vi "Begin.vi"(8 "error in":errorcluster) -> (0 "error out":errorcluster)   [LabVIEW 2018]
doc: "Called before other user functions, this VI is expected to open initial I/O refnums, load in file data, and do all program initialization. Notice that the <B>error out</B> terminal is simply used for data flow. Wiring it to other structures or subVIs ensures that this VI runs first."
uses:
  <vilib>/Rock Robotics/WPI/DriverStation/WPI_DriverStationRobotMode2.ctl
  <vilib>/Rock Robotics/WPI/Joystick/WPI_JoystickDeviceEnum.ctl
  <vilib>/Rock Robotics/WPI/Solenoid/WPI_SolenoidChannel.ctl
  <vilib>/Rock Robotics/WPI/ThirdParty/Phoenix-LabVIEW/Motor Controller/Controls/CTRE_Phoenix_MotorControl_NeutralMode.ctl
  <vilib>/Rock Robotics/WPI/ThirdParty/REV Robotics/SPARK MAX/Typedef/Spark MAX Idle Mode.ctl
  2019 Deep Space Beta/Robot Global Data.vi
  <vilib>/Rock Robotics/Network Tables/NT Write String Array.vi
  <vilib>/Rock Robotics/WPI/Solenoid/WPI_SolenoidOpenDouble.vi
  <vilib>/Rock Robotics/WPI/Solenoid/WPI_SolenoidOpenSingle.vi
  <vilib>/Rock Robotics/WPI/Utilities/WPI_GetSetVariantRefNum.vi
  <vilib>/Rock Robotics/WPI/SerialPort/WPI_SerialPort.ctl
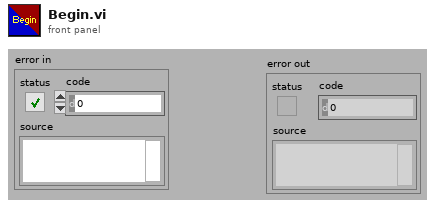
[diagram p1: front panel]
types:
  T1 = typedef "Spark MAX Idle Mode.ctl" = enum16{"Coast", "Brake"}
  T2 = typedef "CTRE_Phoenix_MotorControl_NeutralMode.ctl" = enum8{"EEPROMSetting", "Override to Coast", "Override to Brake"}
  T3 = typedef "WPI_SolenoidChannel.ctl" = enum8{"Solenoid 0", "Solenoid 1", "Solenoid 2", "Solenoid 3", "Solenoid 4", "Solenoid 5", "Solenoid 6", "Solenoid 7", "Invalid"}
  T4 = typedef "WPI_JoystickDeviceEnum.ctl" = enum16{"USB 0", "USB 1", "USB 2", "USB 3", "USB 4", "USB 5"}
  T5 = typedef "WPI_DriverStationRobotMode2.ctl" = enum16{"Autonomous Disabled", "Autonomous Enabled", "Teleop Disabled", "Teleop Enabled", "Disconnected", "Finish", "Test Disabled", "Test Enabled", "Emergency Stopped"}
  T6 = typedef "WPI_JoystickDevRef.ctl" = cluster{"Device":T4}
  T7 = typedef "WPI_MotorControlDeviceRef.ctl" = cluster{"DeviceStatus":errorcluster, "Type":T8, "PWM":cluster{"PWM Channel":T9, "DeadBand":T10}, "CAN":cluster{"Device Number":u8, "SetOutput VI Ref":variant, "GetOutput VI Ref":variant, "Enable VI Ref":variant, "Disable VI Ref":variant, "Data":variant}, "Invert":bool, "DIO PWM":cluster{"PWM \"Enable\" Channel":T9, "DIOChannel":T11, "PWM Rate":dbl}}
  T8 = typedef "WPI_MotorControlType.ctl" = enum16{"PWM", "CAN", "DIO PWM"}
  T9 = typedef "FPGA_DIOPWMChannel.ctl" = enum8{"PWM 0", "PWM 1", "PWM 2", "PWM 3", "PWM 4", "PWM 5", "PWM 6", "PWM 7", "PWM 8", "PWM 9", "PWM MXP 0", "PWM MXP 1", "PWM MXP 2", "PWM MXP 3", "PWM MXP 4", "PWM MXP 5", "PWM MXP 6", "PWM MXP 7", "PWM MXP 8", "PWM MXP 9", "Invalid"}
  T10 = typedef "WPI_PWMDeadband.ctl" = cluster{"Name":string, "maxPositivePwm":i32, "minPositivePwm":i32, "centerPwm":i32, "maxNegativePwm":i32, "minNegativePwm":i32, "angularRange":u16}
  T11 = typedef "FPGA_DIOChannel.ctl" = enum8{"DIO 0", "DIO 1", "DIO 2", "DIO 3", "DIO 4", "DIO 5", "DIO 6", "DIO 7", "DIO 8", "DIO 9", "DIO MXP 0", "DIO MXP 1", "DIO MXP 2", "DIO MXP 3", "DIO MXP 4", "DIO MXP 5", "DIO MXP 6", "DIO MXP 7", "DIO MXP 8", "DIO MXP 9", "DIO MXP 10", "DIO MXP 11", "DIO MXP 12", "DIO MXP 13", "DIO MXP 14", "DIO MXP 15", "SPI Port CS1", "SPI Port CS2", "SPI Port CS3", "SPI Port MISO", "SPI Port MOSI", "Invalid"}
  T12 = typedef "WPI_SerialPort.ctl" = enum16{"Onboard RS-232", "MXP TTL", "USB 1", "USB 2"}
  T13 = typedef "WPI_SerialPortRef.ctl" = cluster{"DevStatus":errorcluster, "Serial Port Name":refnum<visa-resource-name>}
  T14 = typedef "WPI_CompressorDevRef.ctl" = cluster{"DevStatus":errorcluster, "Pneumatics Control Module":u8}
  T15 = typedef "WPI_SolenoidDevRef.ctl" = cluster{"DevStatus":errorcluster, "Pneumatics Control Module":u8, "Forward Solenoid Channel":T3, "Reverse Solenoid Channel":T3}
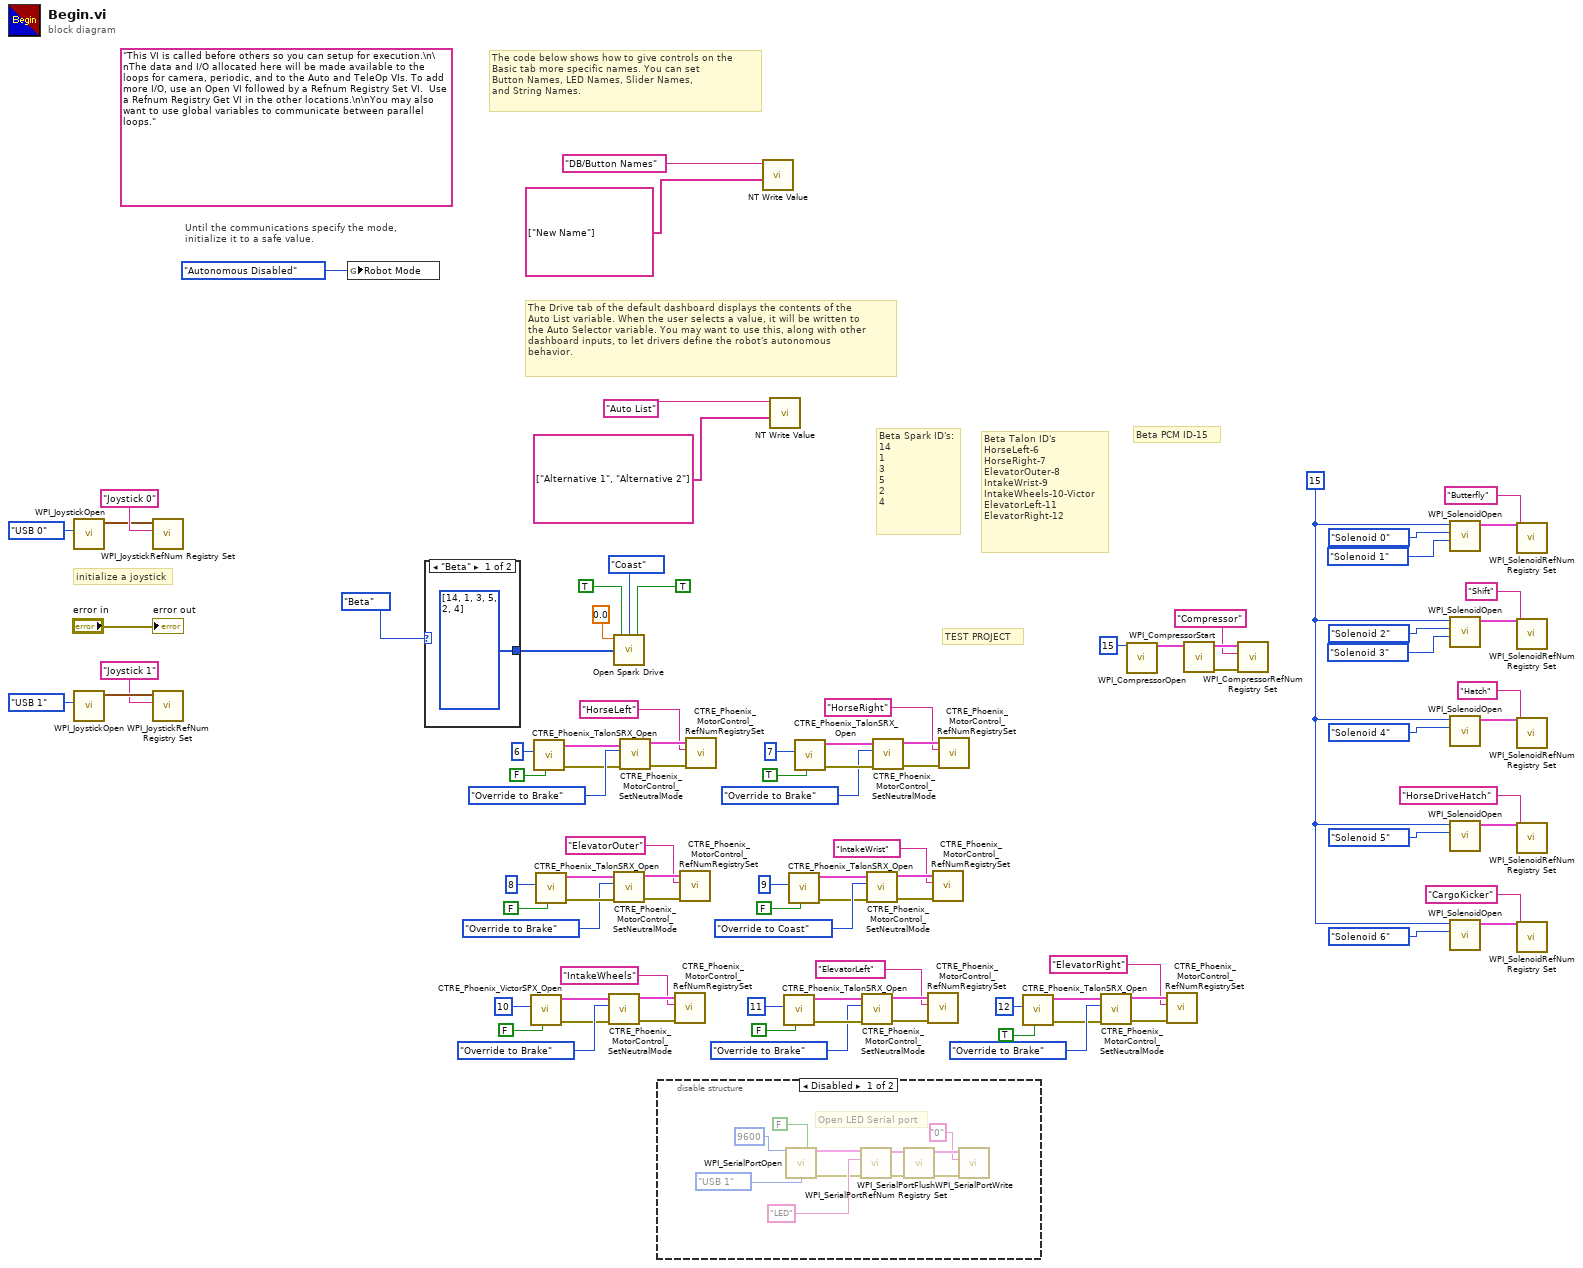
[diagram p0: block diagram]
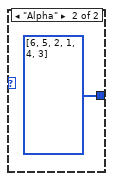
[diagram p2: hidden frame]
diagram:
  w69 = u8 15 ("Pneumatics Control Module (0)")
  (unwired) "This VI is called before others so you can setup for execution.\n\nThe data and I/O allocated here will be made available to the loops for camera, periodic, and to the Auto and TeleOp VIs. To add more I/O, use an Open VI followed by a Refnum Registry Set VI.  Use a Refnum Registry Get VI in the other locations.\n\nYou may also want to use global variables to communicate between parallel loops."
  # "Beta PCM ID-15"
  # "Beta Talon ID's\nHorseLeft-6\nHorseRight-7\nElevatorOuter-8\nIntakeWrist-9\nIntakeWheels-10-Victor\nElevatorLeft-11\nElevatorRight-12"
  # "Beta Spark ID's:\n14\n1\n3\n5\n2\n4"
  # "TEST PROJECT"
  # "The Drive tab of the default dashboard displays the contents of the\nAuto List variable. When the user selects a value, it will be written to\nthe Auto Selector variable. You may want to use this, along with other\ndashboard inputs, to let drivers define the robot's autonomous\nbehavior."
  # "The code below shows how to give controls on the\nBasic tab more specific names. You can set\nButton Names, LED Names, Slider Names,\nand String Names."
  # "initialize a joystick"
  # "Until the communications specify the mode,\ninitialize it to a safe value."
  n1 = call <vilib>:"WPI_JoystickOpen.vi"("JoystickDevice"=WPI_JoystickDeviceEnum."USB 0") -> ("JoystickDevRef"=w95:T6)  [unwired: 10 in]
  n2 = call <vilib>:"WPI_JoystickOpen.vi"("JoystickDevice"=WPI_JoystickDeviceEnum."USB 1") -> ("JoystickDevRef"=w87:T6)  [unwired: 10 in]
  n3 = call <vilib>:"WPI_JoystickRefNum Registry Set.vi"("refnum name"="Joystick 0", "JoystickDevRef"=w95) -> ()  [unwired: 8 in, 2 out]
  n4 = call <vilib>:"WPI_JoystickRefNum Registry Set.vi"("refnum name"="Joystick 1", "JoystickDevRef"=w87) -> ()  [unwired: 8 in, 2 out]
  n5 = global write "Robot Global Data.vi" "Robot Mode"(WPI_DriverStationRobotMode2."Autonomous Disabled" ("Robot Mode")) -> ()
  n6 = case shown="\"Beta\"" enum16{"Alpha", "Beta"}."Beta" {
    tunnel: [u8[] [14, 1, 3, 5, 2, 4] ("CAN IDs") u8[] [6, 5, 2, 1, 4, 3] ("CAN IDs")] -> w1
    frame "Beta" {
    }
    frame "Alpha" {
    }
  }
  n7 = call <vilib>:"CTRE_Phoenix_VictorSPX_Open.vi"("Invert"=FALSE, "Device Number"=u8 10) -> ("error out"=w50:errorcluster, "CAN Talon SRX Ref"=w51:T7)  [unwired: 8 in]
  n8 = call <vilib>:"CTRE_Phoenix_TalonSRX_Open.vi"("Invert"=FALSE, "Device Number"=u8 6) -> ("error out"=w16:errorcluster, "CAN Talon SRX Ref"=w17:T7)  [unwired: 8 in]
  n9 = call <vilib>:"CTRE_Phoenix_TalonSRX_Open.vi"("Invert"=FALSE, "Device Number"=u8 8) -> ("error out"=w55:errorcluster, "CAN Talon SRX Ref"=w54:T7)  [unwired: 8 in]
  n10 = call <vilib>:"CTRE_Phoenix_MotorControl_SetNeutralMode.vi"("error in (no error)"=w50, "Motor Control Neutral Mode"=CTRE_Phoenix_MotorControl_NeutralMode."Override to Brake", "PhoenixMotorControlDevRef"=w51) -> ("error out"=w48:errorcluster, "PhoenixMotorControlDevRef"=w49:T7)  [unwired: 7 in]
  n11 = call "Open Spark Drive.vi"("Set Master/Slave?"=TRUE, "Set Ramp Rate?"=TRUE, "CAN IDs"=w1, "Idle Mode"=Spark_MAX_Idle_Mode."Coast", "Full Acceleration Time"=sgl 0.0 ("Seconds from neutral to full (0)")) -> ()  [unwired: 7 in]
  n12 = call <vilib>:"CTRE_Phoenix_MotorControl_SetNeutralMode.vi"("error in (no error)"=w55, "Motor Control Neutral Mode"=CTRE_Phoenix_MotorControl_NeutralMode."Override to Brake", "PhoenixMotorControlDevRef"=w54) -> ("error out"=w57:errorcluster, "PhoenixMotorControlDevRef"=w56:T7)  [unwired: 7 in]
  n13 = call <vilib>:"CTRE_Phoenix_MotorControl_SetNeutralMode.vi"("error in (no error)"=w16, "Motor Control Neutral Mode"=CTRE_Phoenix_MotorControl_NeutralMode."Override to Brake", "PhoenixMotorControlDevRef"=w17) -> ("error out"=w60:errorcluster, "PhoenixMotorControlDevRef"=w61:T7)  [unwired: 7 in]
  n14 = disable-structure shown="Disabled" {
    frame Disabled {
      # "Open LED Serial port"
      n15 = call <vilib>:"WPI_SerialPortOpen.vi"("Baud Rate"=u32 9600, "Enable Termination Char? (T)"=FALSE, "Serial Port"=WPI_SerialPort."USB 1") -> ("SerialPortRef"=w108:T13, "error out"=w106:errorcluster)  [unwired: 11 in]
      n16 = call <vilib>:"WPI_SerialPortRefNum Registry Set.vi"("error in (no error)"=w106, "refnum name"="LED", "SerialPortRef"=w108) -> ("error out"=w102:errorcluster, "SerialPortRef"=w103:T13)  [unwired: 7 in]
      n17 = call <vilib>:"WPI_SerialPortFlush.vi"("error in (no error)"=w102, "SerialPortRef"=w103) -> ("error out"=w105:errorcluster, "SerialPortRef"=w104:T13)  [unwired: 8 in]
      n18 = call <vilib>:"WPI_SerialPortWrite.vi"("error in (no error)"=w105, "Buffer"="0", "SerialPortRef"=w104) -> ()  [unwired: 6 in, 3 out]
    }
    frame Enabled {
    }
  }
  n19 = call <vilib>:"CTRE_Phoenix_MotorControl_RefNumRegistrySet.vi"("error in (no error)"=w48, "refnum name"="IntakeWheels" ("string"), "PhoenixMotorControlDevRef"=w49) -> ()  [unwired: 7 in, 2 out]
  n20 = call <vilib>:"CTRE_Phoenix_MotorControl_RefNumRegistrySet.vi"("error in (no error)"=w57, "refnum name"="ElevatorOuter" ("string"), "PhoenixMotorControlDevRef"=w56) -> ()  [unwired: 7 in, 2 out]
  n21 = call <vilib>:"CTRE_Phoenix_MotorControl_RefNumRegistrySet.vi"("error in (no error)"=w60, "refnum name"="HorseLeft" ("string"), "PhoenixMotorControlDevRef"=w61) -> ()  [unwired: 7 in, 2 out]
  n22 = call-poly <vilib>:"NT Write Value.vi"("String Array"=string[] ["New Name"], "Name"="DB/Button Names") -> ()  [unwired: 9 in, 1 out]
  n23 = call-poly <vilib>:"NT Write Value.vi"("String Array"=string[] ["Alternative 1", "Alternative 2"], "Name"="Auto List") -> ()  [unwired: 9 in, 1 out]
  n24 = call <vilib>:"CTRE_Phoenix_TalonSRX_Open.vi"("Invert"=FALSE, "Device Number"=u8 11) -> ("error out"=w41:errorcluster, "CAN Talon SRX Ref"=w40:T7)  [unwired: 8 in]
  n25 = call <vilib>:"CTRE_Phoenix_TalonSRX_Open.vi"("Invert"=FALSE, "Device Number"=u8 9) -> ("error out"=w36:errorcluster, "CAN Talon SRX Ref"=w37:T7)  [unwired: 8 in]
  n26 = call <vilib>:"CTRE_Phoenix_TalonSRX_Open.vi"("Invert"=TRUE, "Device Number"=u8 7) -> ("error out"=w27:errorcluster, "CAN Talon SRX Ref"=w26:T7)  [unwired: 8 in]
  n27 = call <vilib>:"CTRE_Phoenix_MotorControl_SetNeutralMode.vi"("error in (no error)"=w41, "Motor Control Neutral Mode"=CTRE_Phoenix_MotorControl_NeutralMode."Override to Brake", "PhoenixMotorControlDevRef"=w40) -> ("error out"=w43:errorcluster, "PhoenixMotorControlDevRef"=w42:T7)  [unwired: 7 in]
  n28 = call <vilib>:"CTRE_Phoenix_MotorControl_SetNeutralMode.vi"("error in (no error)"=w36, "Motor Control Neutral Mode"=CTRE_Phoenix_MotorControl_NeutralMode."Override to Coast", "PhoenixMotorControlDevRef"=w37) -> ("error out"=w34:errorcluster, "PhoenixMotorControlDevRef"=w35:T7)  [unwired: 7 in]
  n29 = call <vilib>:"CTRE_Phoenix_MotorControl_SetNeutralMode.vi"("error in (no error)"=w27, "Motor Control Neutral Mode"=CTRE_Phoenix_MotorControl_NeutralMode."Override to Brake", "PhoenixMotorControlDevRef"=w26) -> ("error out"=w29:errorcluster, "PhoenixMotorControlDevRef"=w28:T7)  [unwired: 7 in]
  n30 = call <vilib>:"CTRE_Phoenix_MotorControl_RefNumRegistrySet.vi"("error in (no error)"=w43, "refnum name"="ElevatorLeft" ("string"), "PhoenixMotorControlDevRef"=w42) -> ()  [unwired: 7 in, 2 out]
  n31 = call <vilib>:"CTRE_Phoenix_MotorControl_RefNumRegistrySet.vi"("error in (no error)"=w34, "refnum name"="IntakeWrist" ("string"), "PhoenixMotorControlDevRef"=w35) -> ()  [unwired: 7 in, 2 out]
  n32 = call <vilib>:"CTRE_Phoenix_MotorControl_RefNumRegistrySet.vi"("error in (no error)"=w29, "refnum name"="HorseRight" ("string"), "PhoenixMotorControlDevRef"=w28) -> ()  [unwired: 7 in, 2 out]
  n33 = call <vilib>:"CTRE_Phoenix_TalonSRX_Open.vi"("Invert"=TRUE, "Device Number"=u8 12) -> ("error out"=w22:errorcluster, "CAN Talon SRX Ref"=w23:T7)  [unwired: 8 in]
  n34 = call <vilib>:"CTRE_Phoenix_MotorControl_SetNeutralMode.vi"("error in (no error)"=w22, "Motor Control Neutral Mode"=CTRE_Phoenix_MotorControl_NeutralMode."Override to Brake", "PhoenixMotorControlDevRef"=w23) -> ("error out"=w20:errorcluster, "PhoenixMotorControlDevRef"=w21:T7)  [unwired: 7 in]
  n35 = call <vilib>:"WPI_CompressorOpen.vi"("Pneumatics Control Module (0)"=u8 15) -> ("CompressorDevRef"=w67:T14)  [unwired: 13 in, 1 out]
  n36 = call <vilib>:"CTRE_Phoenix_MotorControl_RefNumRegistrySet.vi"("error in (no error)"=w20, "refnum name"="ElevatorRight" ("string"), "PhoenixMotorControlDevRef"=w21) -> ()  [unwired: 7 in, 2 out]
  n37 = call <vilib>:"WPI_CompressorStart.vi"("CompressorDevRef"=w67) -> ("error out"=w65:errorcluster, "CompressorDevRef"=w64:T14)  [unwired: 9 in]
  n38 = call <vilib>:"WPI_CompressorRefNum Registry Set.vi"("error in (no error)"=w65, "refnum name"="Compressor", "CompressorDevRef"=w64) -> ()  [unwired: 7 in, 2 out]
  n39 = call-poly <vilib>:"WPI_SolenoidOpen.vi"("Reverse Solenoid Channel"=WPI_SolenoidChannel."Solenoid 1", "Forward Solenoid Channel"=WPI_SolenoidChannel."Solenoid 0", "Pneumatics Control Module (0)"=w69) -> ("SolenoidDevRef"=w85:T15)  [unwired: 7 in, 1 out]
  n40 = call-poly <vilib>:"WPI_SolenoidOpen.vi"("Reverse Solenoid Channel"=WPI_SolenoidChannel."Solenoid 3", "Forward Solenoid Channel"=WPI_SolenoidChannel."Solenoid 2", "Pneumatics Control Module (0)"=w69) -> ("SolenoidDevRef"=w79:T15)  [unwired: 7 in, 1 out]
  n41 = call-poly <vilib>:"WPI_SolenoidOpen.vi"("Solenoid Channel"=WPI_SolenoidChannel."Solenoid 4" ("Forward Solenoid Channel"), "Pneumatics Control Module (0)"=w69) -> ("SolenoidDevRef"=w78:T15)  [unwired: 8 in, 1 out]
  n42 = call-poly <vilib>:"WPI_SolenoidOpen.vi"("Solenoid Channel"=WPI_SolenoidChannel."Solenoid 5" ("Forward Solenoid Channel"), "Pneumatics Control Module (0)"=w69) -> ("SolenoidDevRef"=w73:T15)  [unwired: 8 in, 1 out]
  n43 = call-poly <vilib>:"WPI_SolenoidOpen.vi"("Solenoid Channel"=WPI_SolenoidChannel."Solenoid 6" ("Forward Solenoid Channel"), "Pneumatics Control Module (0)"=w69) -> ("SolenoidDevRef"=w72:T15)  [unwired: 8 in, 1 out]
  n44 = call <vilib>:"WPI_SolenoidRefNum Registry Set.vi"("refnum name"="Butterfly", "SolenoidDevRef"=w85) -> ()  [unwired: 8 in, 2 out]
  n45 = call <vilib>:"WPI_SolenoidRefNum Registry Set.vi"("refnum name"="Shift", "SolenoidDevRef"=w79) -> ()  [unwired: 8 in, 2 out]
  n46 = call <vilib>:"WPI_SolenoidRefNum Registry Set.vi"("refnum name"="Hatch", "SolenoidDevRef"=w78) -> ()  [unwired: 8 in, 2 out]
  n47 = call <vilib>:"WPI_SolenoidRefNum Registry Set.vi"("refnum name"="HorseDriveHatch", "SolenoidDevRef"=w73) -> ()  [unwired: 8 in, 2 out]
  n48 = call <vilib>:"WPI_SolenoidRefNum Registry Set.vi"("refnum name"="CargoKicker", "SolenoidDevRef"=w72) -> ()  [unwired: 8 in, 2 out]
  "error out" <- "error in"
